vi "Main v0.81.vi"() -> ()   [LabVIEW 2017]
doc: "v0.5:\n\n- Added Reject to Manual Mode\n- Send reject pallet cluster during manual mode\n- Run continuous manual happens only when no error has occured"
uses:
  Controls/Main Tabs.ctl
  Controls/Auto.ctl
  RT/Controls/Auto Delays.ctl
  RT/Controls/Auto Times.ctl
  Controls/UI Data.ctl
  support/Message Queue/Enqueue Message (Single).vi
  <vilib>/Utility/error.llb/Error Cluster From Error Code.vi
  <vilib>/ErrorRing/Error Ring.xnode
  support/Message Queue/Message Queue.lvlib
  support/User Event - Stop/User Event - Stop.lvlib
panel:
  out "Date-Time":string caption="Dip-Tube Assembly Automation (HMI) v0.8"
  out "Main Tab":T1
  in  "Autocycle":T2
  in  "Manual":bool
  in  "Parameters":bool
  in  "Maintenance":bool
  in  "Save Para":bool
  in  "Home Para":bool
  in  "ParaTab":T3(tab)
  in  "StopperRearDelay":dbl format="%#.2f"
  in  "StopperFrontDelay":dbl format="%#.2f"
  in  "MaxAlarms":dbl caption="Max Alarms in 1 Minute" format="%#.2f"
  in  "MaxConsecutive":dbl caption="Max Consecutive Alarms" format="%#.2f"
  in  "Gate Close Delay":dbl format="%#.2f"
  in  "Gate Open Delay":dbl format="%#.2f"
  in  "BF Off Delay":dbl format="%#.2f"
  in  "BF On Delay":dbl format="%#.2f"
  in  "DelayAfterReject":dbl format="%#.2f"
  in  "MeasurementTime":dbl format="%#.2f"
  in  "DelayAfterMesFront":dbl format="%#.2f"
  in  "DelayAfterCut":dbl format="%#.2f"
  in  "DelayAfterCutClamp":dbl format="%#.2f"
  in  "DelayAfterInsClamp":dbl format="%#.2f"
  in  "DelayToClose":dbl format="%#.2f"
  in  "DelayToOpen":dbl format="%#.2f"
  in  "DelayAfterInsertion":dbl format="%#.2f"
  in  "DelayBeforeInsertion":dbl format="%#.2f"
  in  "AgitatorUpTime":dbl format="%#.2f"
  in  "AgitatorDownTime":dbl format="%#.2f"
  in  "Reset MCount":bool
  in  "Enable BF?":bool
  in  "Enable Agitate?":bool
  in  "Reject Pallets":T4
  in  "Enable Reject?":bool
  in  "Toggle Motor":bool
  in  "Continuous?":bool
  in  "Enable Measure?":bool
  in  "Enable Index?":bool
  in  "Enable PF?":bool
  in  "Auto Delays":T5={"Agitator Delays"=[400, 250], "TF Delays"=[700, 800, 2], "Insertion Delays"=[100, 500], "Cutting Delays"=[300, 300, 100], "PF Delays"=[250, 30000], "Measur. Delays"=[500], "Reject Delays"=[500], "BF Delays"=[1000, 1000]}
  in  "Enable Cutting?":bool
  in  "Enable Insertion?":bool
  in  "Run Manual":bool
  in  "Enable TF?":bool
  in  "Home Manual":bool
  out "Status":T7
  out "Measurements":T8 {"Height 1" format="%#.2f"; "Height 2" format="%#.2f"; "Height 3" format="%#.2f"; "Height 4" format="%#.2f"}
  out "OutputCount":u32
  in  "All IO":bool
  in  "Stats":bool
  in  "Home AC":bool
  out "Status":string
  out "Count":dbl format="%06.0f"
  out "Count 3":dbl caption="Cycle Time" format="%0.2f"
  out "Count 2":dbl caption="Rejects" format="%06.0f"
  in  "Statuses":string[][](table)
  in  "Exit":bool
  # "Vision Harmony Dip-Tube Assembly Automation"
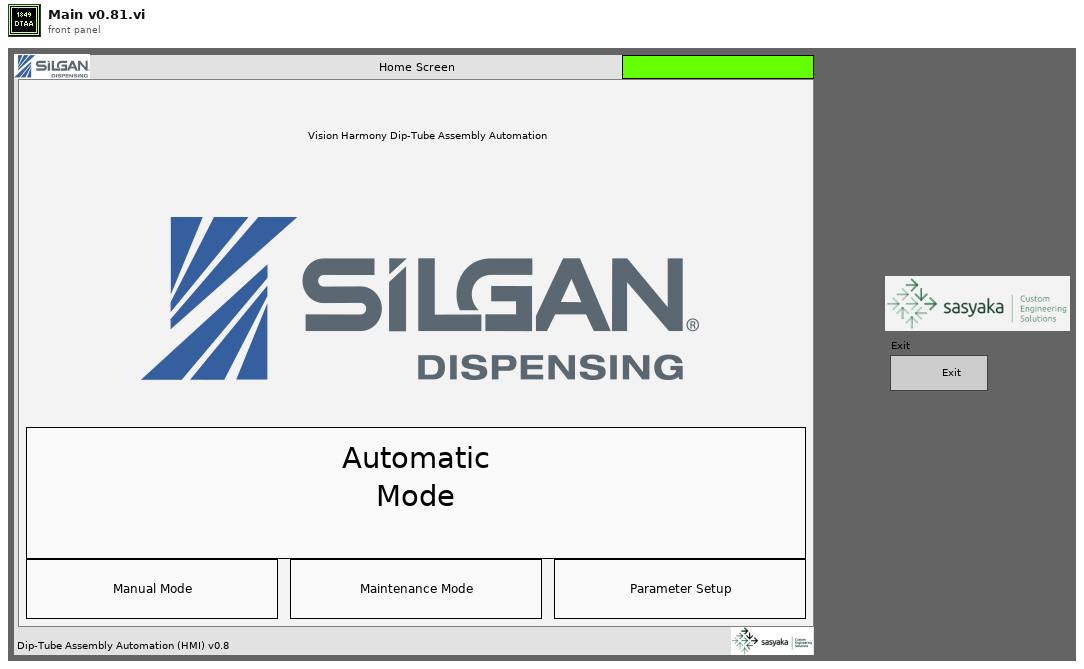
[diagram p1: front panel]
types:
  T1 = typedef "Main Tabs.ctl" = enum32{"Home Screen", "Parameter Setup", "Manual Mode", "Autocycle"}
  T2 = typedef "Auto.ctl" = bool
  T3 = enum32{"General & Indexing", "Bowl Feeder & Pump Conveyor", "Cutting, Measurement & Rejection", "Tube Feeder & Insertion"}
  T4 = cluster{"Reject 1":bool, "Reject 2":bool, "Reject 3":bool, "Reject 4":bool}
  T5 = typedef "Auto Delays.ctl" = cluster{"Agitator Delays":u32[], "TF Delays":u32[], "Insertion Delays":u32[], "Cutting Delays":u32[], "PF Delays":u32[], "Measur. Delays":u32[], "Reject Delays":u32[], "BF Delays":u32[]}
  T6 = typedef "Auto Times.ctl" = cluster{"Index Time":u32, "TF Time":u32, "Insertion Time":u32, "Cutting Time":u32, "PF Time":u32, "Meas. Time":u32, "Reject Time":u32}
  T7 = cluster{"Auto Times":T6, "error out":errorcluster}
  T8 = cluster{"Height 1":dbl, "Height 2":dbl, "Height 3":dbl, "Height 4":dbl}
  T9 = typedef "UI Data.ctl" = cluster{"Main Tab":refnum<vi>}
  T10 = typedef "Message Queue.lvlib/All Message Queues.ctl" = cluster{"UI":refnum<queue>}
  T11 = enum8{"Enabled", "Disabled", "Disabled and Grayed Out"}
  T12 = cluster{"Auto Times":T6, "Measurements":cluster{"1":dbl, "2":dbl, "3":dbl, "4":dbl}, "OutputCount":u32, "error out":errorcluster}
  T13 = cluster{"Auto Delays":T5, "Reject Pallets":cluster{"Reject 1":bool, "Reject 2":bool, "Reject 3":bool, "Reject 4":bool}}
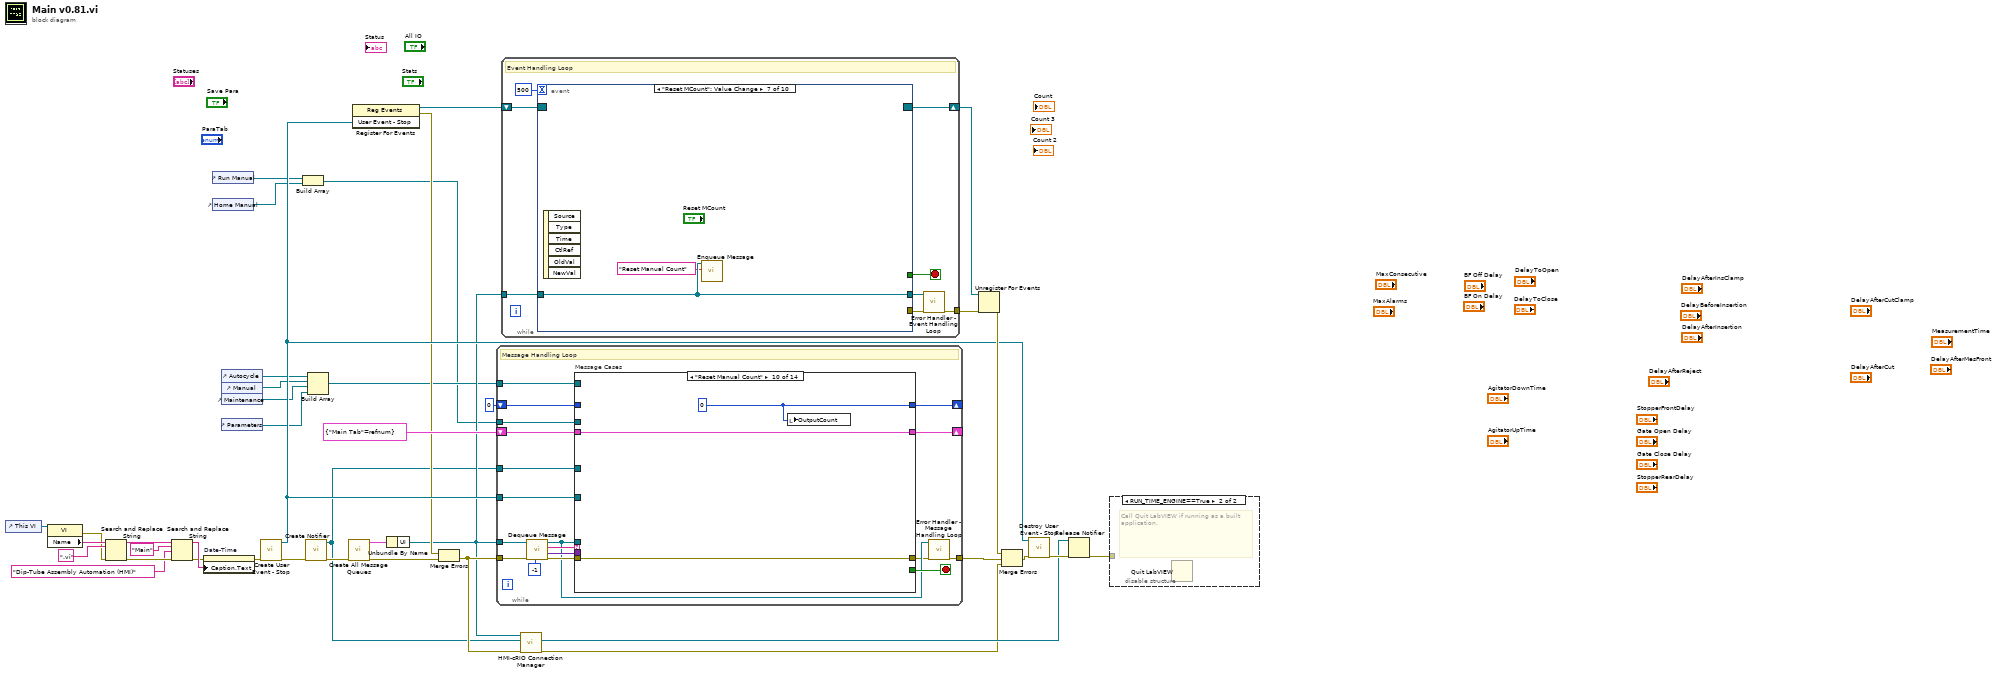
[diagram p0: block diagram]
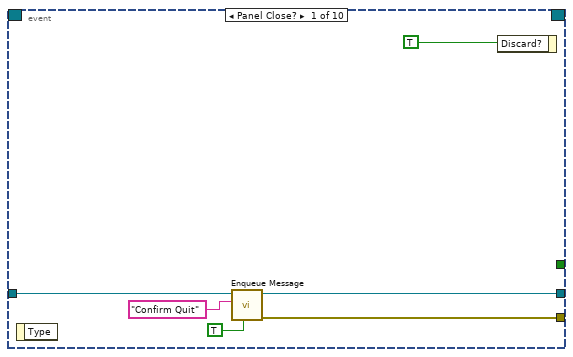
[diagram p2: hidden frame]
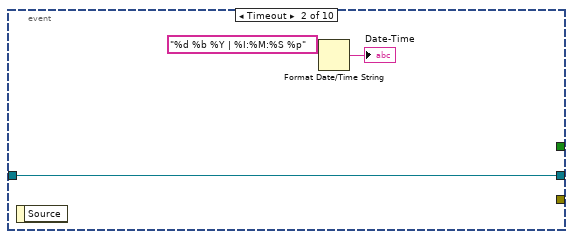
[diagram p3: hidden frame]
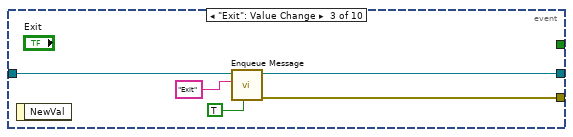
[diagram p4: hidden frame]
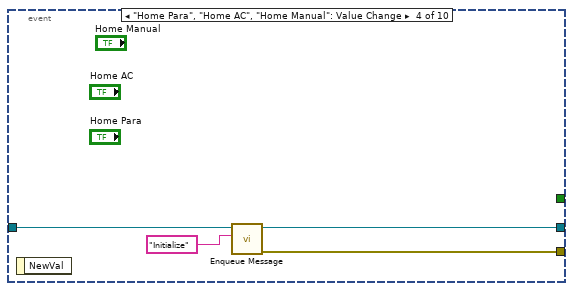
[diagram p5: hidden frame]
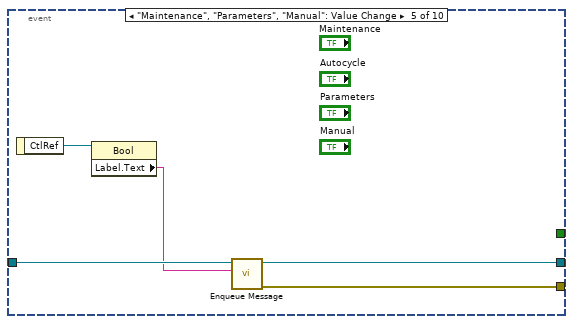
[diagram p6: hidden frame]
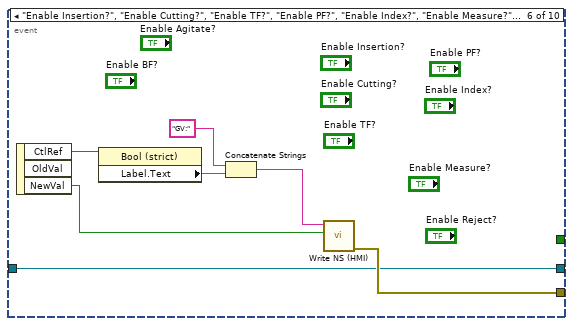
[diagram p7: hidden frame]
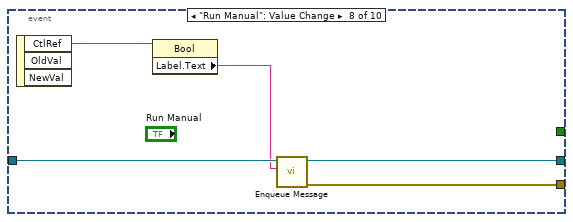
[diagram p8: hidden frame]
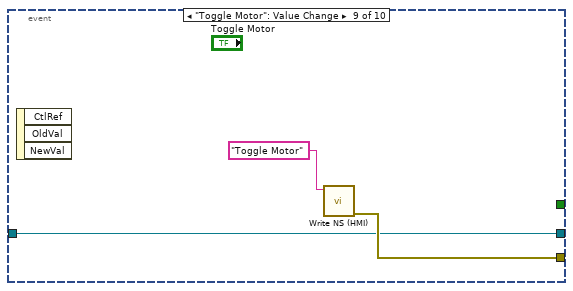
[diagram p9: hidden frame]
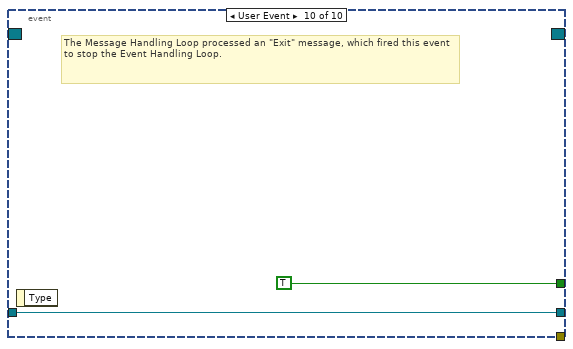
[diagram p10: hidden frame]
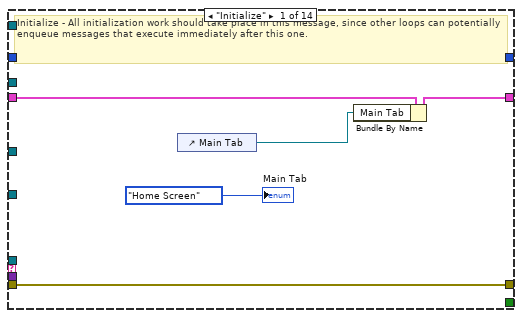
[diagram p11: hidden frame]
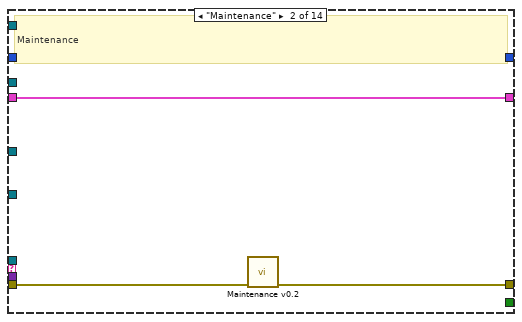
[diagram p12: hidden frame]
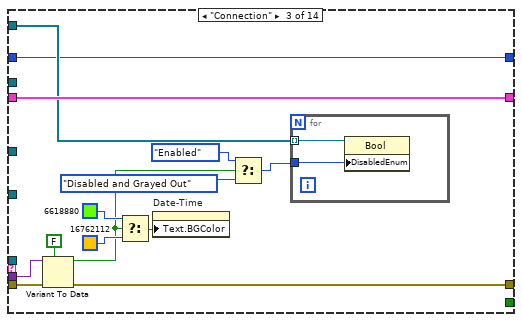
[diagram p13: hidden frame]
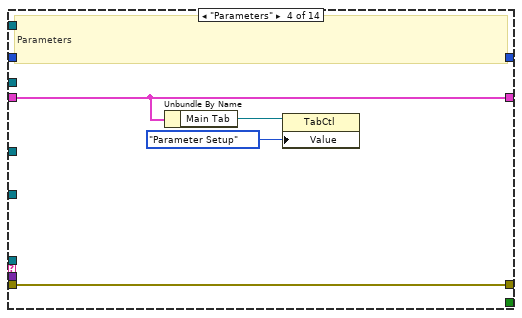
[diagram p14: hidden frame]
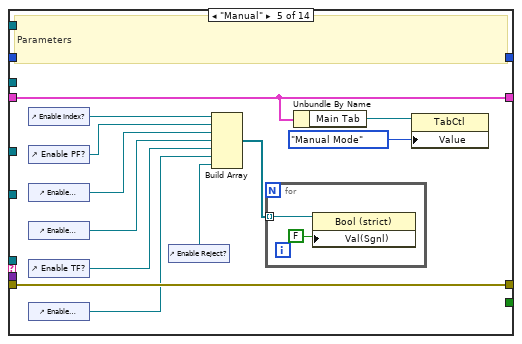
[diagram p15: hidden frame]
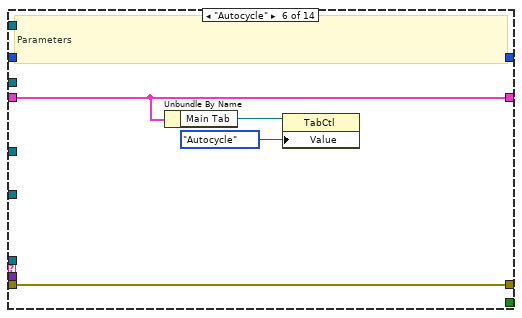
[diagram p16: hidden frame]
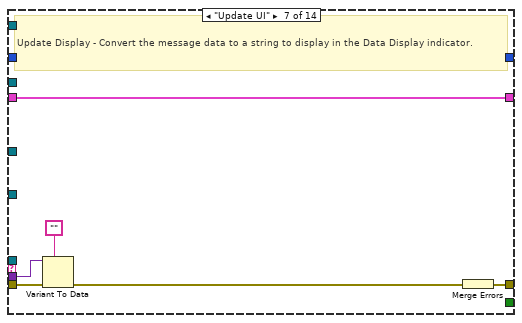
[diagram p17: hidden frame]
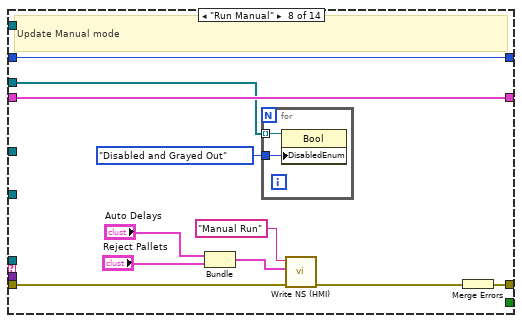
[diagram p18: hidden frame]
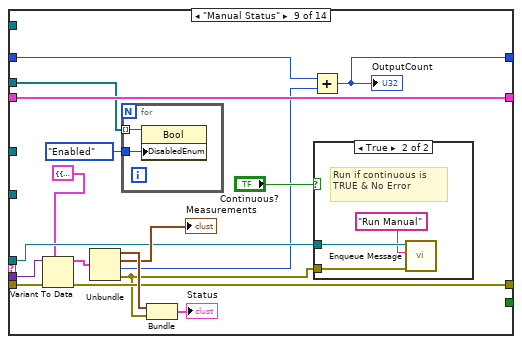
[diagram p19: hidden frame]
diagram:
  n1 = control-ref of="This VI"() -> (w9:refnum<vi>)
  n2 = property class="VI"(reference=w9) -> (error out=w8:errorcluster, "Name"=w15:string)  [unwired: 1 in, 1 out]
  n3 = Search and Replace String(input string=w15, search string=".vi", error in=w8) -> (result string=w13:string, error out=w12:errorcluster)  [unwired: 5 in, 2 out]
  n4 = Search and Replace String(input string=w13, search string="Main", replace string="Dip-Tube Assembly Automation (HMI)" ("replace string (\"\")"), error in=w12) -> (result string=w7:string, error out=w6:errorcluster)  [unwired: 4 in, 2 out]
  n5 = property on="Date-Time" class="Str"(error in=w6, "Caption.Text"=w7) -> (error out=w5:errorcluster)  [unwired: 1 in, 1 out]
  n6 = control-ref of="Run Manual"() -> (w4:refnum<vi>)
  n7 = control-ref of="Home Manual"() -> (w3:refnum<vi>)
  n8 = control-ref of="Autocycle"() -> (w20:refnum<vi>)
  n9 = control-ref of="Manual"() -> (w19:refnum<vi>)
  n10 = control-ref of="Maintenance"() -> (w18:refnum<vi>)
  n11 = control-ref of="Parameters"() -> (w17:refnum<vi>)
  n12 = call "Create User Event - Stop.vi"("error in (no error)"=w5) -> ("error out"=w27:errorcluster, "User Event - Stop"=w31:refnum<user-event>)  [unwired: 9 in]
  n13 = Build Array(w4, w3) -> (w2:refnum<vi>[])
  n14 = call "Create Notifier.vi"("error in (no error)"=w27) -> ("error out"=w26:errorcluster, "notifier out"=w21:refnum<notifier>)  [unwired: 9 in]
  n15 = Build Array(w20, w19, w18, w17) -> (w16:refnum<vi>[])
  n16 = call "Create All Message Queues.vi"("error in (no error)"=w26) -> ("error out"=w40:errorcluster, "Message Queues out"=w39:T10)  [unwired: 9 in]
  n17 = register-events(w31) -> (reference out=w32:refnum<event-registration>, error out=w30:errorcluster)  [unwired: 2 in]
  n18 = Unbundle By Name(w39) -> ("UI"=w28:refnum<queue>)
  n19 = Merge Errors(w30, w40) -> (w29:errorcluster)
  n20 = while {
    tunnel: w28 -> [w50]
    shift-right: [w57] -> _
    shift-left: T9 {"Main Tab"=refnum} ("Data Cluster") -> [w58]
    tunnel: w31 -> [w55]
    tunnel: w29 -> [w54]
    tunnel: [w48] -> w38
    tunnel: w21 -> [w45]
    tunnel: w16 -> [w44]
    tunnel: w2 -> [w43]
    shift-right: [w41] -> _
    shift-left: u32 0 ("OutputCount") -> [w42]
    stop <- w56 stop-if-true
    # "Message Handling Loop"
    n21 = call "Dequeue Message.vi"("timeout"=-1, "error in (no error)"=w54, "Message Queue"=w50) -> ("error out"=w53:errorcluster, "Message Data"=w51:variant, "Message"=w52:string, "dup Message Queue"=w49:refnum<queue>)  [unwired: 5 in]
    n22 = case "Message Cases" shown="\"Reset Manual Count\"" w52 {
      selector: w52 -> [_ _ _ _ _ _ _ _ _ _ _ _ _ w187]
      tunnel: w49 -> [_ _ _ _ _ _ _ _ w136 _ _ w166 w185 _]
      tunnel: w53 -> [w64 w67 w80 w89 w102 w109 w114 w124 w145 w154 w162 w170 w178 _]
      tunnel: [w64 w66 w79 w89 w102 w109 w115 w126 w135 w154 w156 w168 w181 w188] -> w47
      tunnel: w58 -> [w63 w68 w82 w88 w101 w108 w116 w127 w146 w153 w161 w169 w184 w189]
      tunnel: [w62 w68 w82 w88 w101 w108 w116 w127 w146 w153 w161 w169 w184 w189] -> w57
      tunnel: [_ _ _ _ _ _ _ _ _ _ _ _ TRUE _] -> w56
      tunnel: w51 -> [_ _ w78 _ _ _ w113 _ w144 _ w160 _ w175 _]
      tunnel: w55 -> [_ _ _ _ _ _ _ _ _ _ _ _ w180 _]
      tunnel: w45 -> [_ _ _ _ _ _ _ _ _ _ _ _ w174 _]
      tunnel: w44 -> [_ _ w74 _ _ _ _ _ _ _ _ _ _ _]
      tunnel: w43 -> [_ _ _ _ _ _ _ w121 w142 _ _ _ _ _]
      tunnel: w42 -> [w59 w65 w69 w85 w90 w105 w110 w117 w132 _ w155 w163 w171 w186]
      tunnel: [w59 w65 w69 w85 w90 w105 w110 w117 w131 w152 w155 w163 w171 w186] -> w41
      frame "Initialize" {
        # "Initialize - All initialization work should take place in this message, since other loops can potentially enqueue messages that execute immediately after this one."
        n23 = control-ref of="Main Tab"() -> (w61:refnum<vi>)
        n24 = Bundle By Name(cluster=w63, "Main Tab"=w61) -> (w62:T9)
        "Main Tab" <- Main_Tabs."Home Screen" ("Main Tab")
      }
      frame "Maintenance" {
        # "Maintenance"
        n25 = call "Maintenance v0.2.vi"("Error In"=w67) -> ("Error out"=w66:errorcluster)  [unwired: 10 in]
      }
      frame "Connection" {
        n26 = Variant To Data(error in=w80, type=FALSE, Variant=w78) -> (data=w73:bool, error out=w79:errorcluster)
        n27 = Select(t=u32 6618880 ("Text.Text Colors:BG Color"), s=w73, f=u32 16762112 ("Text.Text Colors:BG Color")) -> (s? t:f=w75:u32)
        n28 = property on="Date-Time" class="Str"("Text.BGColor"=w75) -> ()  [unwired: 2 in, 2 out]
        n29 = Select(t=T11."Enabled" ("Disabled"), s=w73, f=T11."Disabled and Grayed Out") -> (s? t:f=w71:T11)
        n30 = for {
          tunnel: w74 -> [w84] mode=indexing
          tunnel: w71 -> [w83]
          n31 = property class="Bool"(reference=w84, "DisabledEnum"=w83) -> ()  [unwired: 1 in, 2 out]
        }
      }
      frame "Parameters" {
        # "Parameters"
        n32 = Unbundle By Name(w88) -> ("Main Tab"=w87:refnum<vi>)
        n33 = property class="TabCtl"(reference=w87, "Value"=Main_Tabs."Parameter Setup" ("Main Tab")) -> ()  [unwired: 1 in, 2 out]
      }
      frame "Manual" {
        # "Parameters"
        n34 = control-ref of="Enable Index?"() -> (w98:refnum<vi>)
        n35 = control-ref of="Enable PF?"() -> (w97:refnum<vi>)
        n36 = control-ref of="Enable Cutting?"() -> (w96:refnum<vi>)
        n37 = control-ref of="Enable Insertion?"() -> (w95:refnum<vi>)
        n38 = control-ref of="Enable TF?"() -> (w94:refnum<vi>)
        n39 = control-ref of="Enable Measure?"() -> (w92:refnum<vi>)
        n40 = control-ref of="Enable Reject?"() -> (w91:refnum<vi>)
        n41 = Build Array(w98, w97, w96, w95, w94, w92, w91) -> (w93:refnum<vi>[])
        n42 = for {
          tunnel: w93 -> [w104] mode=indexing
          n43 = property class="Bool (strict)"(reference=w104, "Val(Sgnl)"=FALSE ("Value (Signaling)")) -> ()  [unwired: 1 in, 2 out]
        }
        n44 = Unbundle By Name(w101) -> ("Main Tab"=w100:refnum<vi>)
        n45 = property class="TabCtl"(reference=w100, "Value"=Main_Tabs."Manual Mode" ("Main Tab")) -> ()  [unwired: 1 in, 2 out]
      }
      frame "Autocycle" {
        # "Parameters"
        n46 = Unbundle By Name(w108) -> ("Main Tab"=w107:refnum<vi>)
        n47 = property class="TabCtl"(reference=w107, "Value"=Main_Tabs."Autocycle" ("Main Tab")) -> ()  [unwired: 1 in, 2 out]
      }
      frame "Update UI" {
        # "Update Display - Convert the message data to a string to display in the Data Display indicator."
        n48 = Variant To Data(error in=w114, type="", Variant=w113) -> (error out=w111:errorcluster)  [unwired: 1 out]
        n49 = Merge Errors(w111) -> (w115:errorcluster)
      }
      frame "Run Manual" {
        # "Update Manual mode"
        n50 = Bundle("Auto Delays"="Auto Delays", "Reject Pallets"="Reject Pallets") -> (w118:T13)  [unwired: 1 in]
        n51 = for {
          tunnel: w121 -> [w129] mode=indexing
          tunnel: T11."Disabled and Grayed Out" ("Disabled") -> [w128]
          n52 = property class="Bool"(reference=w129, "DisabledEnum"=w128) -> ()  [unwired: 1 in, 2 out]
        }
        n53 = call "Write NS (HMI).vi"("error in (no error)"=w124, "Message Data"=w118, "Message"="Manual Run") -> ("error out"=w123:errorcluster)  [unwired: 8 in]
        n54 = Merge Errors(w123) -> (w126:errorcluster)
      }
      frame "Manual Status" {
        n55 = Variant To Data(error in=w145, type=T12 {"Auto Times"={"Index Time"=0, "TF Time"=0, "Insertion Time"=0, "Cutting Time"=0, "PF Time"=0, "Meas. Time"=0, "Reject Time"=0}, "Measurements"={"1"=0.0, "2"=0.0, "3"=0.0, "4"=0.0}, "OutputCount"=0, "error out"={"status"=FALSE, "code"=0, "source"=""}} ("cluster"), Variant=w144) -> (data=w141:T12, error out=w135:errorcluster)
        n56 = Unbundle(w141) -> ("Auto Times"=w140:T6, "Measurements"=→"Measurements":cluster{"1":dbl, "2":dbl, "3":dbl, "4":dbl}, "OutputCount"=w133:u32, "error out"=w130:errorcluster)
        n57 = for {
          tunnel: w142 -> [w151] mode=indexing
          tunnel: T11."Enabled" ("Disabled") -> [w150]
          n58 = property class="Bool"(reference=w151, "DisabledEnum"=w150) -> ()  [unwired: 1 in, 2 out]
        }
        n59 = Bundle("Auto Times"=w140, "error out"=w130) -> (→"Status":T7)  [unwired: 1 in]
        n60 = Add(x=w132, y=w133) -> (x+y=w131:u32)
        "OutputCount" <- w131
        n61 = case shown="True" "Continuous?" {
          tunnel: w136 -> [_ w149]
          tunnel: w130 -> [_ w148]
          frame False {
          }
          frame True {
            # "Run if continuous is TRUE & No Error"
            n62 = call-poly "Enqueue Message.vi"("error in (no error)"=w148, "Message"="Run Manual", "Message Queue"=w149) -> ()  [unwired: 7 in, 2 out]
          }
        }
      }
      frame "Reset Manual Count" {
        w152 = u32 0 ("OutputCount")
        n63 = local write "OutputCount"(w152) -> ()
      }
      frame "Error" {
        # "Error - Display an error dialog. This message is sent by the \"Error Handler\" VIs at the end of other loops in this application."
        n64 = Variant To Data(error in=w162, type=errorcluster {"status"=FALSE, "code"=0, "source"=""} ("error constant"), Variant=w160) -> (data=w158:errorcluster, error out=w157:errorcluster)
        n65 = call <vilib>:"Simple Error Handler.vi"("error in (no error)"=w158) -> ()  [unwired: 4 in, 5 out]
        n66 = Merge Errors(w157) -> (w156:errorcluster)
      }
      frame "Confirm Quit" {
        # "Confirm Quit - Message that can confirm whether or not the user wants to exit the application."
        n67 = call-poly "Enqueue Message.vi"("Priority Message? (F)"=TRUE, "error in (no error)"=w170, "Message"="Exit", "Message Queue"=w166) -> ("error out"=w167:errorcluster)  [unwired: 6 in, 1 out]
        n68 = Merge Errors(w167) -> (w168:errorcluster)
      }
      frame "Exit" {
        # "Stop the VI"
        # "Release the message queue reference"
        # "Exit - Exit the application."
        n69 = Variant To Data(type=errorcluster {"status"=FALSE, "code"=0, "source"=""} ("error constant"), Variant=w175) -> (data=w176:errorcluster)  [unwired: 1 in, 1 out]
        n70 = call <vilib>:"Simple Error Handler.vi"("error in (no error)"=w176) -> ()  [unwired: 4 in, 5 out]
        n71 = Send Notification(notification=TRUE, notifier=w174) -> (error out=w172:errorcluster)  [unwired: 1 in, 1 out]
        n72 = call "Fire User Event - Stop.vi"("User Event - Stop"=w180) -> ("error out"=w179:errorcluster)  [unwired: 10 in]
        n73 = Release Queue(queue=w185, error in (no error)=w178) -> (error out=w182:errorcluster)  [unwired: 1 in, 2 out]
        n74 = Merge Errors(w172, w179, w182) -> (w181:errorcluster)
      }
      frame Default {
        # "'Default' case only runs if there is a message that isn't defined in any of the other cases.  Output a programming error."
        n75 = xnode "Error Ring"("parameter 0"=w187) -> ("error out"=w188:errorcluster)
      }
    }
    n76 = call "Error Handler - Message Handling Loop.vi"("error in (no error)"=w47, "Message Queue"=w49) -> ("dup error in"=w48:errorcluster)  [unwired: 8 in, 1 out]
  }
  n77 = while {
    tunnel: w28 -> [w204]
    shift-right: [w202] -> w35
    shift-left: w32 -> [w203]
    tunnel: [w198] -> w33
    stop <- w200 stop-if-true
    # "Event Handling Loop"
    n78 = event shown="[6] \"Reset MCount\": Value Change" {
      selector: w203 -> [_ _ _ _ _ _ _ _ _ _]
      dyn-events: [_ _ _ _ _ _ _ _ _ _] -> w202
      timeout: 500 -> [_ _ _ _ _ _ _ _ _ _]
      tunnel: [_ _ _ _ _ _ _ _ _ TRUE ("Discard?")] -> w200
      tunnel: w204 -> [w209 w213 w218 w222 w227 w232 w236 w241 w243 w246]
      tunnel: [w208 _ w217 w221 w226 w233 _ w239 w244 _] -> w201
      tunnel: [w207 w213 w216 w220 w225 w232 w236 w240 w243 w246] -> w199
      event Panel Close? {
        n79 = event-data() -> ()  [unwired: 1 in, 1 out]
        n80 = call-poly "Enqueue Message.vi"("Priority Message? (F)"=TRUE, "Message"="Confirm Quit", "Message Queue"=w209) -> ("error out"=w208:errorcluster, "dup Message Queue"=w207:refnum<queue>)  [unwired: 7 in]
        n81 = event-data("Discard?"=TRUE) -> ()  [unwired: 1 in, 1 out]
      }
      event Timeout {
        n82 = event-data() -> ()  [unwired: 1 in, 1 out]
        n83 = Format Date/Time String(time format string (%c)="%d %b %Y | %I:%M:%S %p") -> (date/time string=→"Date-Time":string)  [unwired: 2 in]
      }
      event "Exit": Value Change {
        n84 = event-data() -> ()  [unwired: 1 in, 1 out]
        n85 = call-poly "Enqueue Message.vi"("Priority Message? (F)"=TRUE, "Message"="Exit", "Message Queue"=w218) -> ("error out"=w217:errorcluster, "dup Message Queue"=w216:refnum<queue>)  [unwired: 7 in]
      }
      event "Home Para", "Home AC", "Home Manual": Value Change {
        n86 = event-data() -> ()  [unwired: 1 in, 1 out]
        n87 = call-poly "Enqueue Message.vi"("Message"="Initialize", "Message Queue"=w222) -> ("error out"=w221:errorcluster, "dup Message Queue"=w220:refnum<queue>)  [unwired: 8 in]
      }
      event "Maintenance", "Parameters", "Manual": Value Change {
        n88 = event-data() -> ("CtlRef"=w224:refnum<vi>)  [unwired: 1 in]
        n89 = property class="Bool"(reference=w224) -> ("Label.Text"=w223:string)  [unwired: 1 in, 2 out]
        n90 = call-poly "Enqueue Message.vi"("Message"=w223, "Message Queue"=w227) -> ("error out"=w226:errorcluster, "dup Message Queue"=w225:refnum<queue>)  [unwired: 8 in]
      }
      event "Enable Insertion?", "Enable Cutting?", "Enable TF?", "Enable PF?", "Enable Index?", "Enable Measure?", "Enable Reject?", "Enable Agitate?", "Enable BF?": Value Change {
        n91 = event-data() -> ("CtlRef"=w234:refnum<vi>, "NewVal"=w228:bool)  [unwired: 1 in, 1 out]
        n92 = property class="Bool (strict)"(reference=w234) -> ("Label.Text"=w231:string)  [unwired: 1 in, 2 out]
        n93 = Concatenate Strings("GV:" ("string"), w231) -> (w229:string)
        n94 = call "Write NS (HMI).vi"("Message Data"=w228, "Message"=w229) -> ("error out"=w233:errorcluster)  [unwired: 9 in]
      }
      event "Reset MCount": Value Change {
        n95 = event-data() -> ()  [unwired: 1 in, 6 out]
        n96 = call-poly "Enqueue Message.vi"("Message"="Reset Manual Count", "Message Queue"=w236) -> ()  [unwired: 8 in, 2 out]
      }
      event "Run Manual": Value Change {
        n97 = event-data() -> ("CtlRef"=w238:refnum<vi>)  [unwired: 1 in, 2 out]
        n98 = property class="Bool"(reference=w238) -> ("Label.Text"=w237:string)  [unwired: 1 in, 2 out]
        n99 = call-poly "Enqueue Message.vi"("Message"=w237, "Message Queue"=w241) -> ("error out"=w239:errorcluster, "dup Message Queue"=w240:refnum<queue>)  [unwired: 8 in]
      }
      event "Toggle Motor": Value Change {
        n100 = event-data() -> ()  [unwired: 1 in, 3 out]
        n101 = call "Write NS (HMI).vi"("Message"="Toggle Motor") -> ("error out"=w244:errorcluster)  [unwired: 10 in]
      }
      event User Event {
        # "The Message Handling Loop processed an \"Exit\" message, which fired this event to stop the Event Handling Loop."
        n102 = event-data() -> ()  [unwired: 1 in, 1 out]
      }
    }
    n103 = call "Error Handler - Event Handling Loop.vi"("error in (no error)"=w201, "Message Queue"=w199) -> ("dup error in"=w198:errorcluster)  [unwired: 8 in, 1 out]
  }
  n104 = call "HMI-cRIO Connection Manager.vi"("error in"=w29, "notifier in"=w21, "Queue in"=w28) -> ("error out"=w22:errorcluster, "Notifier out"=w23:refnum<notifier>)  [unwired: 7 in]
  n105 = Unregister For Events(event registration refnum=w35, error in=w33) -> (error out=w36:errorcluster)
  n106 = Merge Errors(w36, w38, w22) -> (w37:errorcluster)
  n107 = call "Destroy User Event - Stop.vi"("error in (no error)"=w37, "User Event - Stop"=w31) -> ("error out"=w25:errorcluster)  [unwired: 9 in]
  n108 = Release Notifier(notifier=w23, error in (no error)=w25) -> (error out=w24:errorcluster)  [unwired: 1 in, 2 out]
  n109 = disable-structure shown="RUN_TIME_ENGINE==True" {
    disable-tunnel: w24 -> [_ _]
    frame condition #0 (active) {
    }
    frame condition #1 {
      # "Call Quit LabVIEW if running as a built application."
      n110 = Quit LabVIEW() -> ()  [unwired: 1 in]
    }
  }
